vi "Send.vi"(7 "Message Priority":T1, 8 "error in (no error)":errorcluster, 11 "Message Transport Queue":refnum<class "Message Transport Queue.lvclass">) -> (0 "error out":errorcluster)   [LabVIEW 2016, in "Stream Mediator.lvlib" / "Read Msg.lvclass"]
doc: "--\nCopyright © 2017 Composed SystemsI All rights reserved.\n\nAuthor: Jon McBee <jon.mcbee@composed.io>\n\nThis library is provided \"AS IS\" ,WITHOUT WARRANTIES OR\nCONDITIONS OF ANY KIND, either express or implied.\n\nComposed Systems -- composed.io\n\nStream 0.0.1.1\nJon McBee - Composed Systems\nCopyright (c) 2017, Composed Systems"
uses:
  <userlib>/Composed Systems/Stream/Mediator/Classes/Websocket Client Handler Actor/Websocket Client Handler Msgs/Read Msg/Read Msg.lvclass
  <userlib>/Composed Systems/Stream/Mediator/Classes/Message Transport Queue/Message Transport Queue.lvclass
  <userlib>/Composed Systems/Stream/Mediator/Classes/Message Transport Interface/Message Priority.ctl
  C:/Program Files (x86)/National Instruments/LabVIEW 2016/user.lib/Composed Systems/Stream/Mediator/Classes/Message Interface/Message Interface.lvclass
  <userlib>/Composed Systems/Stream/Mediator/Classes/Message Transport Interface/Message Transport Interface.lvclass
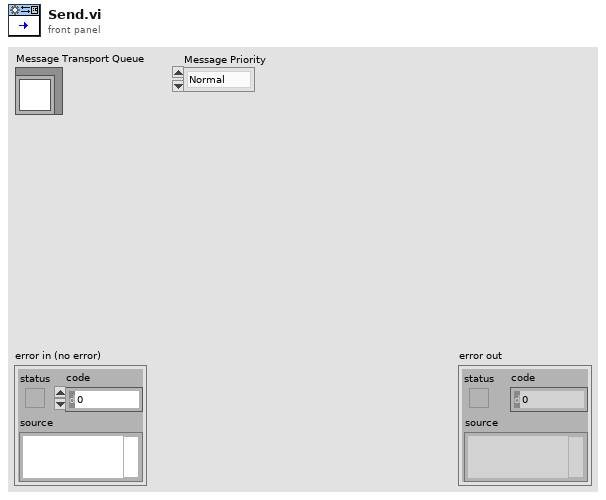
[diagram p1: front panel]
types:
  T1 = typedef "Stream Mediator.lvlib/Message Transport Interface.lvclass/Message Priority.ctl" = enum16{"Normal", "High"}
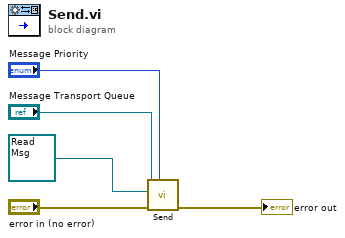
[diagram p0: block diagram]
diagram:
  n1 = call-dynamic "Send.vi"("Message Priority"="Message Priority", "error in (no error)"="error in (no error)", "Message"=refnum<class "Read Msg.lvclass"> refnum ("Read Msg in"), "Message Transport Queue in"="Message Transport Queue") -> ("error out"=→"error out":errorcluster)  [unwired: 5 in, 2 out]
